vi "Open.vi"(8 "error in (no error)":errorcluster, 11 "Device in":refnum<class "Device.lvclass">) -> (0 "error out":errorcluster, 3 "Device out":refnum<class "Device.lvclass">)   [LabVIEW 2020, in "HAL.lvlib" / "Device.lvclass"]
uses:
  Device.lvclass
  Device State.ctl
  <vilib>/Utility/error.llb/Error Cluster From Error Code.vi
  <vilib>/ErrorRing/Error Ring.xnode
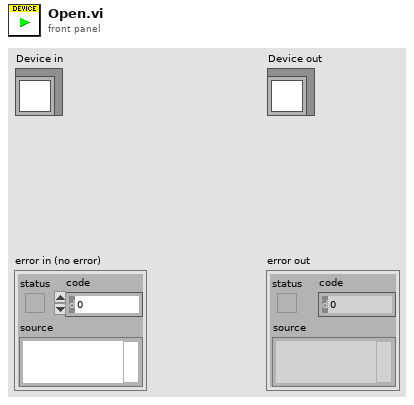
[diagram p1: front panel]
types:
  T1 = typedef "HAL.lvlib/Device.lvclass/Device State.ctl" = enum16{"Uninitialized", "Initialized", "Configured", "Running", "Error"}
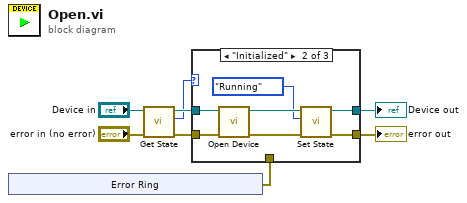
[diagram p0: block diagram]
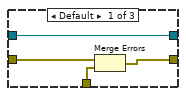
[diagram p2: hidden frame]
diagram:
  n1 = xnode "Error Ring"() -> ("error out"=w1:errorcluster)
  n2 = call "Get State.vi"("error in (no error)"="error in (no error)", "Device in"="Device in") -> ("error out"=w6:errorcluster, "Device State"=w2:T1, "Device out"=w5:refnum<class "Device.lvclass">)  [unwired: 7 in]
  n3 = case shown="\"Initialized\"" w2 {
    tunnel: w6 -> [w11 w18 w20]
    tunnel: w5 -> [w12 w19 w21]
    tunnel: [w12 w15 w21] -> w4
    tunnel: [w10 w14 w20] -> w3
    tunnel: w1 -> [w9 _ _]
    frame Default {
      n4 = Merge Errors(w11, w9) -> (w10:errorcluster)
    }
    frame "Initialized" {
      n5 = call-dynamic "Open Device.vi"("error in (no error)"=w18, "Device in"=w19) -> ("error out"=w17:errorcluster, "Device out"=w16:refnum<class "Device.lvclass">)  [unwired: 8 in]
      n6 = call "Set State.vi"("error in (no error)"=w17, "Device State"=Device_State."Running", "Device in"=w16) -> ("error out"=w14:errorcluster, "Device out"=w15:refnum<class "Device.lvclass">)  [unwired: 7 in]
    }
    frame "Running" {
    }
  }
  "error out" <- w3
  "Device out" <- w4
